vi "DA_NextStep.vi"(8 "error in":errorcluster, 10 "PCtoMyRio":T1={"Command"=enum."End", "Error?"=FALSE, "Stop"=FALSE, "StopPomiar"=FALSE, "Name"="", "FilesPath"=path "", "ErrorHandler"={"Threads"=enum."Acquisistion", "ClearError"=FALSE, "Error Out "={"status"=FALSE, "code"=0, "source"=""}, "Error"=FALSE}, "Fs"=0.0}, 11 "PreviousStep":T4) -> (0 "error out":errorcluster, 3 "NextStep":T4)   [LabVIEW 2019]
uses:
  TypeDef/#TypeDef_EnumOp_DataAcquisition.ctl
  Communication/TypeDef/#TypeDef_FromPCtoMR.ctl
  Communication/TypeDef/#TypeDef_Command.ctl
  Communication/TypeDef/#TypeDef_ErrorHandler_prop.ctl
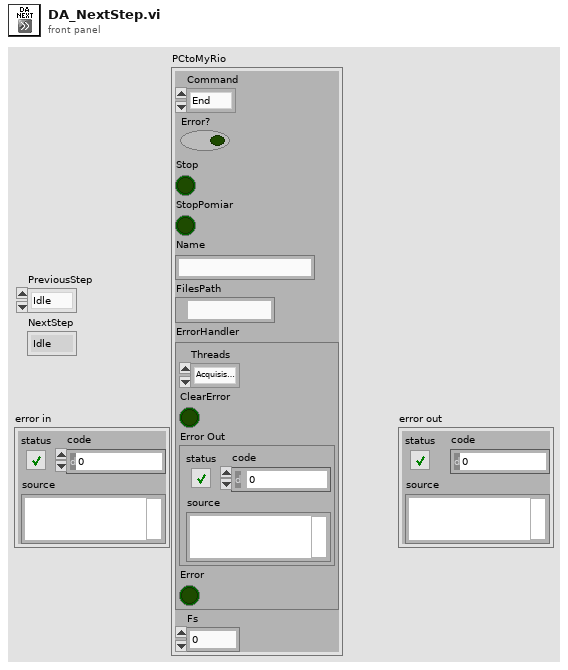
[diagram p1: front panel]
types:
  T1 = typedef "#TypeDef_FromPCtoMR.ctl" = cluster{"Command":T2, "Error?":bool, "Stop":bool, "StopPomiar":bool, "Name":string, "FilesPath":path, "ErrorHandler":T3, "Fs":dbl}
  T2 = typedef "#TypeDef_Command.ctl" = enum16{"Start", "End"}
  T3 = typedef "#TypeDef_ErrorHandler_prop.ctl" = cluster{"Threads":enum16{"Acquisistion", "Data Operation", "Save File"}, "ClearError":bool, "Error Out ":errorcluster, "Error":bool}
  T4 = typedef "#TypeDef_EnumOp_DataAcquisition.ctl" = enum16{"Idle", "Init", "Acq", "End", "Error_Shutdown", "ClearError"}
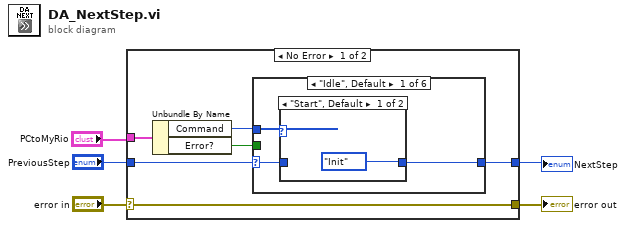
[diagram p0: block diagram]
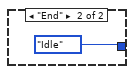
[diagram p2: hidden frame]
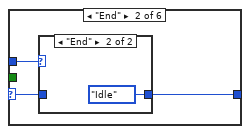
[diagram p3: hidden frame]
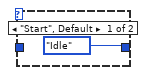
[diagram p4: hidden frame]
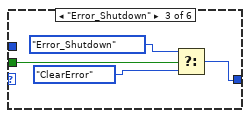
[diagram p5: hidden frame]
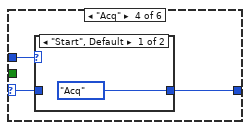
[diagram p6: hidden frame]
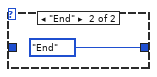
[diagram p7: hidden frame]
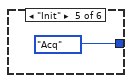
[diagram p8: hidden frame]
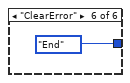
[diagram p9: hidden frame]
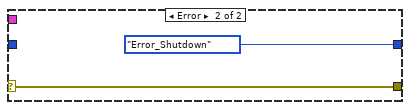
[diagram p10: hidden frame]
diagram:
  n1 = case shown="No Error" "error in" {
    selector: "error in" -> [w10 w34]
    tunnel: [w10 w34] -> w5
    tunnel: [w6 #TypeDef_EnumOp_DataAcquisition."Error_Shutdown" ("PreviousStep 2")] -> w2
    tunnel: "PCtoMyRio" -> [w9 _]
    tunnel: "PreviousStep" -> [w8 _]
    frame No Error {
      n2 = Unbundle By Name(w9) -> ("Command"=w11:T2, "Error?"=w7:bool)
      n3 = case shown="\"Idle\", Default" w8 {
        selector: w8 -> [w13 w18 _ w27 _ _]
        tunnel: w11 -> [w14 w19 _ w26 _ _]
        tunnel: [w12 w17 w24 w28 #TypeDef_EnumOp_DataAcquisition."Acq" ("PreviousStep 2") #TypeDef_EnumOp_DataAcquisition."End" ("PreviousStep 2")] -> w6
        tunnel: w7 -> [_ _ w25 _ _ _]
        frame "Idle", Default {
          n4 = case shown="\"Start\", Default" w14 {
            tunnel: [#TypeDef_EnumOp_DataAcquisition."Init" ("PreviousStep 2") #TypeDef_EnumOp_DataAcquisition."Idle" ("PreviousStep 2")] -> w12
            tunnel: w13 -> [_ _]
            frame "Start", Default {
            }
            frame "End" {
            }
          }
        }
        frame "End" {
          n5 = case shown="\"End\"" w19 {
            tunnel: w18 -> [_ _]
            tunnel: [#TypeDef_EnumOp_DataAcquisition."Idle" ("PreviousStep 2") #TypeDef_EnumOp_DataAcquisition."Idle" ("PreviousStep 2")] -> w17
            frame "Start", Default {
            }
            frame "End" {
            }
          }
        }
        frame "Error_Shutdown" {
          n6 = Select(t=#TypeDef_EnumOp_DataAcquisition."Error_Shutdown" ("PreviousStep 2"), s=w25, f=#TypeDef_EnumOp_DataAcquisition."ClearError" ("PreviousStep 2")) -> (s? t:f=w24:T4)
        }
        frame "Acq" {
          n7 = case shown="\"Start\", Default" w26 {
            tunnel: [#TypeDef_EnumOp_DataAcquisition."Acq" ("PreviousStep 2") #TypeDef_EnumOp_DataAcquisition."End" ("PreviousStep 2")] -> w28
            tunnel: w27 -> [_ _]
            frame "Start", Default {
            }
            frame "End" {
            }
          }
        }
        frame "Init" {
        }
        frame "ClearError" {
        }
      }
    }
    frame Error {
    }
  }
  "error out" <- w5
  "NextStep" <- w2
